vi "CreateEvents_SERVER.vi"(8 "error in (no error)":errorcluster caption="entrée d'erreur (pas d'erreur)", 11 "Control class":refnum<class "Control-Server.lvclass">) -> (0 "error out":errorcluster, 1 "SettingsEventCom":refnum<user-event>, 2 "Event Registration Refnum":refnum<event-registration>, 3 "Control class out":refnum<class "Control-Server.lvclass">)   [LabVIEW 2015]
uses:
  Classes/Control/Control-Server/Control-Server.lvclass
  ControlsVIs/Clusters-def/Message types.ctl
  Classes/Message/Message.lvclass/Message.ctl
  Classes/Message/Message.lvclass
  Classes/GeneralFunctionality/GeneralFunctionality.lvclass
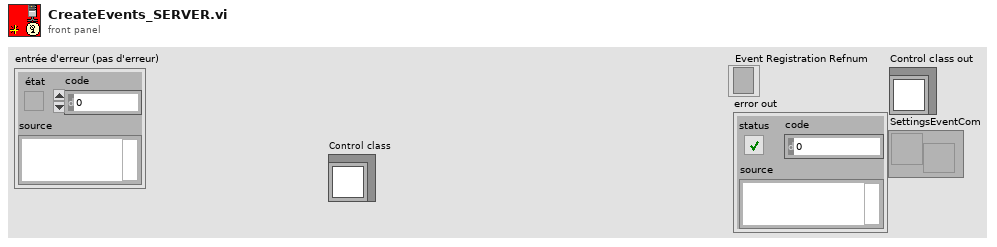
[diagram p1: front panel]
types:
  T1 = typedef "Message types.ctl" = string
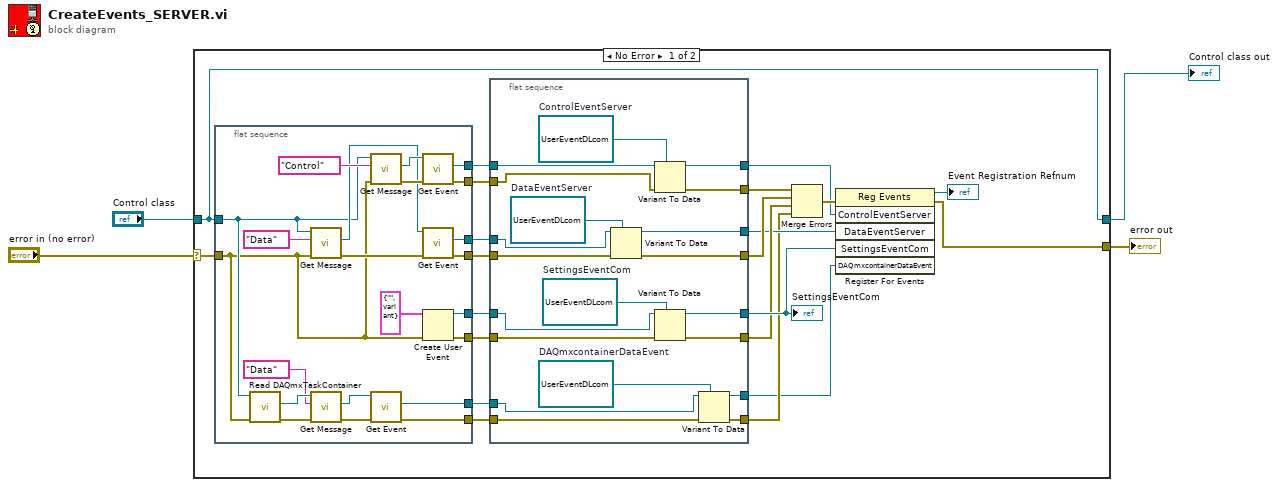
[diagram p0: block diagram]
diagram:
  n1 = case shown="No Error" "error in (no error)" {
    selector: "error in (no error)" -> [w11 w69]
    tunnel: "Control class" -> [w14 w68]
    tunnel: [w25 w69] -> w3
    tunnel: [w14 w68] -> w1
    frame No Error {
      n2 = flat-sequence {
        tunnel: [w65] -> w23
        tunnel: [w64] -> w21
        tunnel: [w62] -> w19
        tunnel: [w61] -> w18
        tunnel: [w59] -> w15
        tunnel: w14 -> [w54]
        tunnel: [w55] -> w13
        tunnel: w11 -> [w53]
        tunnel: [w47] -> w9
        tunnel: [w46] -> w8
        frame #0 {
          n3 = call-dynamic "Read DAQmxTaskContainer.vi"("error in (no error)"=w53, "Control in"=w54) -> ("error out"=w52:errorcluster, "DAQmxTaskContainer.lvclass"=w51:refnum<class "DAQmxTaskContainer.lvclass">)  [unwired: 7 in, 1 out]
          n4 = call "Get Message.vi"("error in (no error)"=w53, "Message type"=T1 "Data", "GeneralFunctionality en entrée"=w54) -> ("error out"=w56:errorcluster, "Message.lvclass"=w58:refnum<class "Message.lvclass">)  [unwired: 6 in, 1 out]
          n5 = call "Get Message.vi"("error in (no error)"=w52, "Message type"=T1 "Data", "GeneralFunctionality en entrée"=w51) -> ("error out"=w49:errorcluster, "Message.lvclass"=w50:refnum<class "Message.lvclass">)  [unwired: 6 in, 1 out]
          n6 = call "Get Message.vi"("error in (no error)"=w53, "Message type"=T1 "Control", "GeneralFunctionality en entrée"=w54) -> ("error out"=w66:errorcluster, "Message.lvclass"=w67:refnum<class "Message.lvclass">)  [unwired: 6 in, 1 out]
          n7 = call "Get Event.vi"("error in (no error)"=w49, "Message en entrée"=w50) -> ("error out"=w46:errorcluster, "UserEventCommand"=w47:refnum<user-event>)  [unwired: 7 in, 1 out]
          n8 = call "Get Event.vi"("error in (no error)"=w66, "Message en entrée"=w67) -> ("error out"=w65:errorcluster, "UserEventCommand"=w64:refnum<user-event>)  [unwired: 7 in, 1 out]
          n9 = call "Get Event.vi"("error in (no error)"=w56, "Message en entrée"=w58) -> ("error out"=w55:errorcluster, "UserEventCommand"=w59:refnum<user-event>)  [unwired: 7 in, 1 out]
          n10 = Create User Event(user event datatype=cluster{"command":string, "data":variant} {"command"="", "data"=variant} ("event data"), error in=w53) -> (user event=w61:refnum<user-event>, error out=w62:errorcluster)
        }
      }
      n11 = flat-sequence {
        tunnel: w23 -> [w45]
        tunnel: [w44] -> w22
        tunnel: w21 -> [w43]
        tunnel: [w42] -> w20
        tunnel: w19 -> [w40]
        tunnel: w18 -> [w39]
        tunnel: [w38] -> w17
        tunnel: [w36] -> w16
        tunnel: w15 -> [w35]
        tunnel: w13 -> [w33]
        tunnel: [w32] -> w12
        tunnel: [w31] -> w10
        tunnel: w9 -> [w27]
        tunnel: w8 -> [w30]
        tunnel: [w29] -> w7
        tunnel: [w26] -> w6
        frame #0 {
          w28 = refnum<user-event> refnum  # DAQmxcontainerDataEvent
          w34 = refnum<user-event> refnum  # DataEventServer
          w37 = refnum<user-event> refnum  # SettingsEventCom
          w41 = refnum<user-event> refnum  # ControlEventServer
          n12 = Variant To Data(error in=w33, type=w34, Variant=w35) -> (data=w31:refnum<user-event>, error out=w32:errorcluster)
          n13 = Variant To Data(error in=w45, type=w41, Variant=w43) -> (data=w42:refnum<user-event>, error out=w44:errorcluster)
          n14 = Variant To Data(error in=w40, type=w37, Variant=w39) -> (data=w38:refnum<user-event>, error out=w36:errorcluster)
          n15 = Variant To Data(error in=w30, type=w28, Variant=w27) -> (data=w26:refnum<user-event>, error out=w29:errorcluster)
        }
      }
      n16 = Merge Errors(w22, w12, w16, w7) -> (w24:errorcluster)
      n17 = register-events(error in=w24, w20, w10, w17, w6) -> (reference out=→"Event Registration Refnum":refnum<event-registration>, error out=w25:errorcluster)  [unwired: 1 in]
      "SettingsEventCom" <- w17
    }
    frame Error {
    }
  }
  "error out" <- w3
  "Control class out" <- w1
